vi "5 Errores.vi"() -> ()   [LabVIEW 2019]
panel:
  in  "Boolean 3":bool
  in  "Boolean 2":bool
  out "Boolean":bool
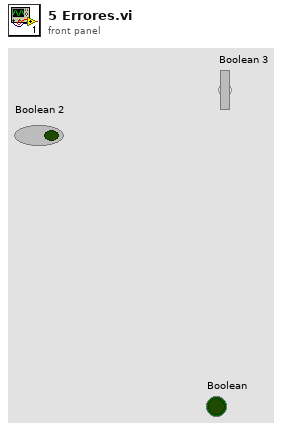
[diagram p1: front panel]
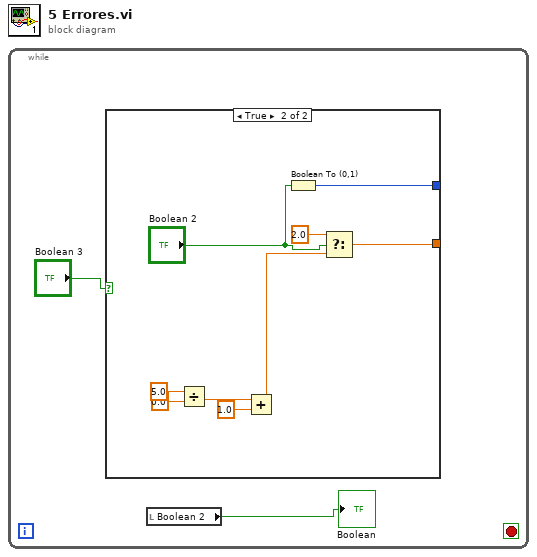
[diagram p0: block diagram]
diagram:
  n1 = while {
    stop <- _ stop-if-true
    n2 = case shown="True" "Boolean 3" {
      tunnel: [_ w6] -> _
      tunnel: [_ w5] -> _
      frame False {
      }
      frame True {
        n3 = Divide(x=5.0, y=0.0) -> (x/y=w9:dbl)
        n4 = Add(x=w9, y=1.0) -> (x+y=w7:dbl)
        n5 = Boolean To (0,1)(Boolean="Boolean 2") -> (0, 1=w5:i16)
        n6 = Select(t=2.0, s="Boolean 2", f=w7) -> (s? t:f=w6:dbl)
      }
    }
    n7 = local read "Boolean 2"() -> (→"Boolean":bool)
  }
